vi "SLM_Camera_Rotatory_MAIN_v2.vi"() -> ()   [LabVIEW 2025]
uses:
  LabVIEW_utils_nick/hologram_states.ctl
  LabVIEW_utils_nick/rotatory_motor_states.ctl
  LabVIEW_utils_nick/states_camera.ctl
panel:
  in  "Fine Tune\nPhase (deg)":dbl=-48.0
  in  "Defocus (mm)":dbl step=1.0
  out "Camera State Queue":refnum<queue>
  out "Motor State Queue":refnum<queue>
  out "SLM State Queue":refnum<queue>
  out "Signal Ready":bool=TRUE
  in  "Pupil Diam. (mm)":dbl=5.6
  in  "Linear Period Y":dbl
  in  "Linear Period X":dbl=-16.0
  in  "SLM Correction":string(combo)="Double-Pass Correction"
  in  "Multipurpose\nCoefficient":dbl
  in  "Eff. Pixel Size":dbl=4.0 step=0.01
  in  "Astigmatism (l)":dbl step=0.01
  in  "Degree Sampling":dbl=1.0
  in  "Calibrate QWP":bool
  in  "N Angles":i16=8 min=8 max=200 step=2
  in  "Measure Stokes":bool
  out "Motor Ready":bool
  in  "Disconnect Motor":bool
  in  "Backward":bool
  in  "Forward":bool
  in  "Motor Name":string="0"
  in  "Encoder Steps/º":i32=398
  in  "Jog Angle (º)":dbl=22.5 format="%#_13g"
  in  "VISA Rotatory Motor":refnum<visa-resource-name>="COM4"
  in  "Connect Motor":bool
  out "SLM Ready":bool=TRUE
  in  "Connect Camera":bool
  in  "View Tab":T1(tab)=enum."Camera Live View"
  out "SLM Display":T2(plugin-control)
  in  "ICImagingControl":refnum<k7>(container)
  out "Snapped Image":T2(plugin-control)
  out "LUT Graph":cluster{dbl[], dbl[]}(graph)={[0.0, 1.0, 2.0, 3.0, 4.0, 5.0, 6.0, 7.0, 8.0, 9.0, 10.0, 11.0, 12.0, 13.0, 14.0, 15.0, 16.0, 17.0, 18.0, 19.0, 20.0, 21.0, 22.0, 23.0, 24.0, 25.0, 26.0, 27.0, 28.0, 29.0, 30.0, 31.0, 32.0, 33.0, 34.0, 35.0, 36.0, 37.0, 38.0, 39.0, 40.0, 41.0, 42.0, 43.0, 44.0, 45.0, 46.0, 47.0, 48.0, 49.0, 50.0, 51.0, 52.0, 53.0, 54.0, 55.0, 56.0, 57.0, 58.0, 59.0, 60.0, 61.0, 62.0, 63.0, 64.0, 65.0, 66.0, 67.0, 68.0, 69.0, 70.0, 71.0, 72.0, 73.0, 74.0, 75.0, 76.0, 77.0, 78.0, 79.0, 80.0, 81.0, 82.0, 83.0, 84.0, 85.0, 86.0, 87.0, 88.0, 89.0, 90.0, 91.0, 92.0, 93.0, 94.0, 95.0, 96.0, 97.0, 98.0, 99.0, 100.0, 101.0, 102.0, 103.0, 104.0, 105.0, 106.0, 107.0, 108.0, 109.0, 110.0, 111.0, 112.0, 113.0, 114.0, 115.0, 116.0, 117.0, 118.0, 119.0, 120.0, 121.0, 122.0, 123.0, 124.0, 125.0, 126.0, 127.0, 128.0, 129.0, 130.0, 131.0, 132.0, 133.0, 134.0, 135.0, 136.0, 137.0, 138.0, 139.0, 140.0, 141.0, 142.0, 143.0, 144.0, 145.0, 146.0, 147.0, 148.0, 149.0, 150.0, 151.0, 152.0, 153.0, 154.0, 155.0, 156.0, 157.0, 158.0, 159.0, 160.0, 161.0, 162.0, 163.0, 164.0, 165.0, 166.0, 167.0, 168.0, 169.0, 170.0, 171.0, 172.0, 173.0, 174.0, 175.0, 176.0, 177.0, 178.0, 179.0, 180.0, 181.0, 182.0, 183.0, 184.0, 185.0, 186.0, 187.0, 188.0, 189.0, 190.0, 191.0, 192.0, 193.0, 194.0], [0.0, 0.010256410256410256, 0.020512820512820513, 0.030769230769230767, 0.041025641025641026, 0.05128205128205128, 0.061538461538461535, 0.07179487179487179, 0.08205128205128205, 0.0923076923076923, 0.10256410256410256, 0.11282051282051282, 0.12307692307692307, 0.13333333333333333, 0.14358974358974358, 0.15384615384615383, 0.1641025641025641, 0.17435897435897432, 0.1846153846153846, 0.19487179487179487, 0.20512820512820512, 0.21538461538461537, 0.22564102564102564, 0.2358974358974359, 0.24615384615384614, 0.2564102564102564, 0.26666666666666666, 0.27692307692307694, 0.28717948717948716, 0.2974358974358974, 0.30769230769230765, 0.31794871794871793, 0.3282051282051282, 0.3384615384615384, 0.34871794871794864, 0.358974358974359, 0.3692307692307692, 0.37948717948717947, 0.38974358974358975, 0.4, 0.41025641025641024, 0.42051282051282046, 0.43076923076923074, 0.441025641025641, 0.4512820512820513, 0.4615384615384615, 0.4717948717948718, 0.48205128205128206, 0.4923076923076923, 0.5025641025641026, 0.5128205128205128, 0.5230769230769231, 0.5333333333333333, 0.5435897435897435, 0.5538461538461539, 0.5641025641025641, 0.5743589743589743, 0.5846153846153845, 0.5948717948717948, 0.6051282051282051, 0.6153846153846153, 0.6256410256410256, 0.6358974358974359, 0.6461538461538462, 0.6564102564102564, 0.6666666666666666, 0.6769230769230768, 0.6871794871794871, 0.6974358974358973, 0.7076923076923077, 0.717948717948718, 0.7282051282051282, 0.7384615384615384, 0.7487179487179487, 0.7589743589743589, 0.7692307692307692, 0.7794871794871795, 0.7897435897435897, 0.8, 0.8102564102564103, 0.8205128205128205, 0.8307692307692307, 0.8410256410256409, 0.8512820512820511, 0.8615384615384615, 0.8717948717948718, 0.882051282051282, 0.8923076923076922, 0.9025641025641026, 0.9128205128205128, 0.923076923076923, 0.9333333333333332, 0.9435897435897436, 0.9538461538461539, 0.9641025641025641, 0.9743589743589743, 0.9846153846153846, 0.9948717948717948, 1.005128205128205, 1.0153846153846153, 1.0256410256410255, 1.035897435897436, 1.0461538461538462, 1.0564102564102564, 1.0666666666666667, 1.0769230769230769, 1.087179487179487, 1.0974358974358973, 1.1076923076923078, 1.117948717948718, 1.1282051282051282, 1.1384615384615384, 1.1487179487179486, 1.1589743589743589, 1.169230769230769, 1.1794871794871793, 1.1897435897435895, 1.2, 1.2102564102564102, 1.2205128205128204, 1.2307692307692306, 1.241025641025641, 1.2512820512820513, 1.2615384615384615, 1.2717948717948717, 1.282051282051282, 1.2923076923076924, 1.3025641025641024, 1.3128205128205128, 1.323076923076923, 1.3333333333333333, 1.3435897435897437, 1.3538461538461537, 1.3641025641025641, 1.3743589743589741, 1.3846153846153846, 1.3948717948717946, 1.405128205128205, 1.4153846153846155, 1.4256410256410255, 1.435897435897436, 1.446153846153846, 1.4564102564102563, 1.4666666666666666, 1.4769230769230768, 1.4871794871794872, 1.4974358974358974, 1.5076923076923077, 1.5179487179487179, 1.528205128205128, 1.5384615384615383, 1.5487179487179488, 1.558974358974359, 1.5692307692307692, 1.5794871794871794, 1.5897435897435896, 1.6, 1.61025641025641, 1.6205128205128205, 1.6307692307692305, 1.641025641025641, 1.6512820512820514, 1.6615384615384614, 1.6717948717948719, 1.6820512820512818, 1.6923076923076923, 1.7025641025641023, 1.7128205128205127, 1.723076923076923, 1.7333333333333332, 1.7435897435897436, 1.7538461538461536, 1.764102564102564, 1.7743589743589743, 1.7846153846153845, 1.7948717948717947, 1.8051282051282052, 1.8153846153846154, 1.8256410256410256, 1.8358974358974358, 1.846153846153846, 1.8564102564102565, 1.8666666666666665, 1.876923076923077, 1.8871794871794871, 1.8974358974358974, 1.9076923076923078, 1.9179487179487178, 1.9282051282051282, 1.9384615384615382, 1.9487179487179487, 1.9589743589743587, 1.9692307692307691, 1.9794871794871796, 1.9897435897435896]}
  out "?":cluster{dbl[], dbl[]}(graph)={[0.0, 1.0, 2.0, 3.0, 4.0, 5.0, 6.0, 7.0, 8.0, 9.0, 10.0, 11.0, 12.0, 13.0, 14.0, 15.0, 16.0, 17.0, 18.0, 19.0, 20.0, 21.0, 22.0, 23.0, 24.0, 25.0, 26.0, 27.0, 28.0, 29.0, 30.0, 31.0, 32.0, 33.0, 34.0, 35.0, 36.0, 37.0, 38.0, 39.0, 40.0, 41.0, 42.0, 43.0, 44.0, 45.0, 46.0, 47.0, 48.0, 49.0, 50.0, 51.0, 52.0, 53.0, 54.0, 55.0, 56.0, 57.0, 58.0, 59.0, 60.0, 61.0, 62.0, 63.0, 64.0, 65.0, 66.0, 67.0, 68.0, 69.0, 70.0, 71.0, 72.0, 73.0, 74.0, 75.0, 76.0, 77.0, 78.0, 79.0, 80.0, 81.0, 82.0, 83.0, 84.0, 85.0, 86.0, 87.0, 88.0, 89.0], [4633679.0, 4655841.0, 4685689.0, 4715698.0, 4744099.0, 4772883.0, 4798670.0, 4826914.0, 4870347.0, 4902083.0, 4922698.0, 4948098.0, 4972552.0, 4995565.0, 5012827.0, 5039209.0, 5052894.0, 5073829.0, 5095346.0, 5114978.0, 5130238.0, 5145058.0, 5165064.0, 5171724.0, 5186128.0, 5187223.0, 5193101.0, 5193411.0, 5194593.0, 5192009.0, 5190420.0, 5184407.0, 5176882.0, 5173530.0, 5161350.0, 5144839.0, 5116936.0, 5111336.0, 5101183.0, 5084166.0, 5070283.0, 5047925.0, 5026346.0, 4999847.0, 4976683.0, 4951600.0, 4928131.0, 4900049.0, 4877127.0, 4851185.0, 4827069.0, 4802488.0, 4781082.0, 4752465.0, 4728072.0, 4703937.0, 4678367.0, 4654771.0, 4629539.0, 4610946.0, 4587405.0, 4565992.0, 4549223.0, 4538346.0, 4521123.0, 4508564.0, 4497075.0, 4492614.0, 4476652.0, 4467015.0, 4463359.0, 4461451.0, 4458074.0, 4459501.0, 4457195.0, 4462532.0, 4470243.0, 4474909.0, 4478224.0, 4493369.0, 4502945.0, 4519712.0, 4534878.0, 4551381.0, 4567135.0, 4590315.0, 4609051.0, 4633947.0, 4651470.0, 4667315.0]}
  in  "Live":bool
  in  "Disconnect Camera":bool
  in  "Camera Properties":bool
  out "Camera Ready":bool
  in  "Grab Image":bool
  in  "Send to SLM":bool=TRUE
  in  "Stop All":bool
  in  "Laser Line (nm)":i32=488
  in  "SLM Cols":i32=1280
  in  "SLM Rows":i32=1024
  in  "Modulation Tab":enum32{"Double Pass", "Single Pass"}(tab)
  in  "Y Offset B":i32 step=1
  in  "Y Offset A":i32 step=1
  in  "X Offset A":i32 step=1
  in  "B Display (Ex)":bool=TRUE
  in  "A Display (Ey)":bool=TRUE
  in  "X Offset B":i32 step=1
  in  "Modulation Mode Double Pass":string(combo)="Laguerre-Gaussian Left"
  in  "Y Offset":i32
  in  "X Offset":i32
  in  "Modulation Type Single Pass":string(combo)="Arrizon Test"
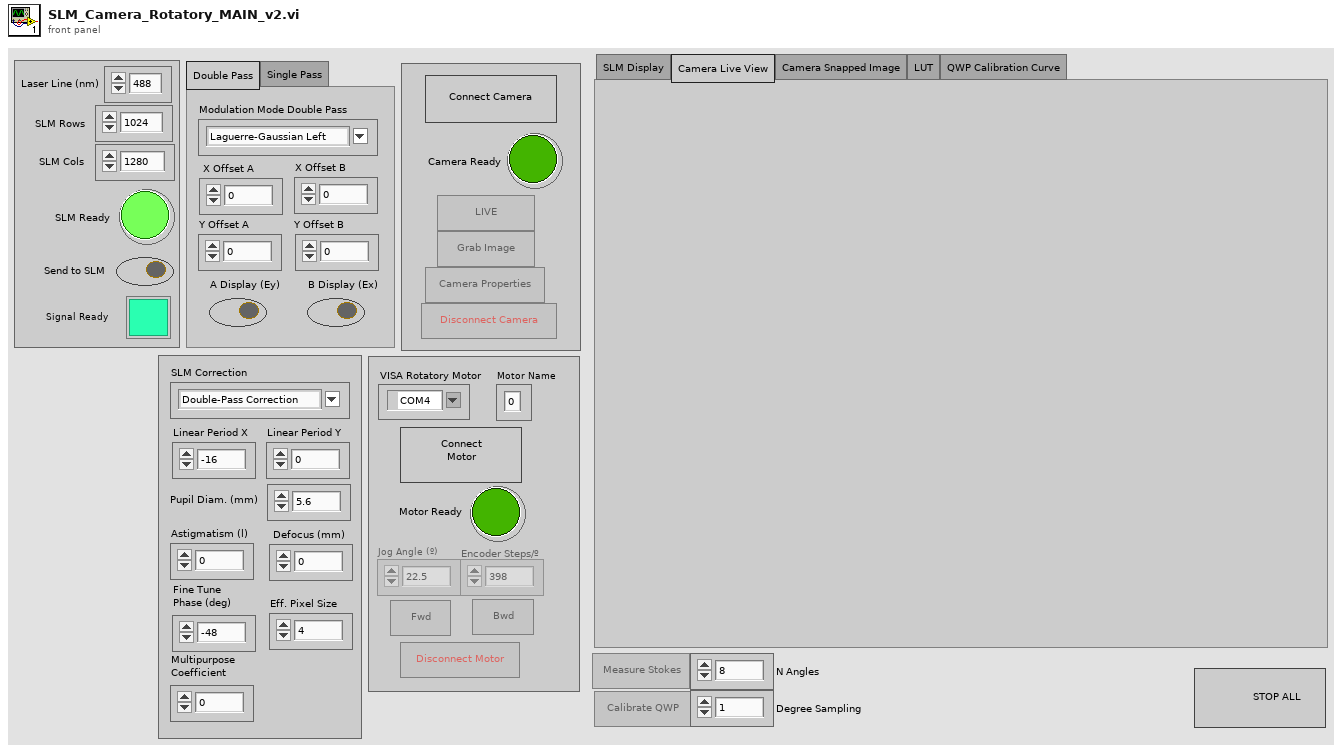
[diagram p1: front panel]
types:
  T1 = enum32{"SLM Display", "Camera Live View", "Camera Snapped Image", "LUT", "QWP Calibration Curve"}
  T2 = typedef "IMAQ Image.ctl" = refnum<image>
  T3 = typedef "rotatory_motor_states.ctl" = enum16{"Set Jog Step", "Move Forward", "Disconnect Motor", "Connect Motor", "Stop All", "Move Backward", "Idle"}
  T4 = typedef "states_camera.ctl" = enum16{"Calibrate QWP Position", "Measure Stokes", "Init Camera", "Idle", "Open Properties", "Grab Image", "Disconnect Camera", "Set Live", "Stop Program", "Calibrate SLM Phase Modulation"}
  T5 = typedef "hologram_states.ctl" = enum16{"Init", "Idle", "Compute Modulation", "Stop All", "Send to SLM"}
  T6 = enum16{"Init", "Idle", "Compute Modulation", "Stop All"}
  T7 = cluster{"status":bool, "code":bool, "source":bool}
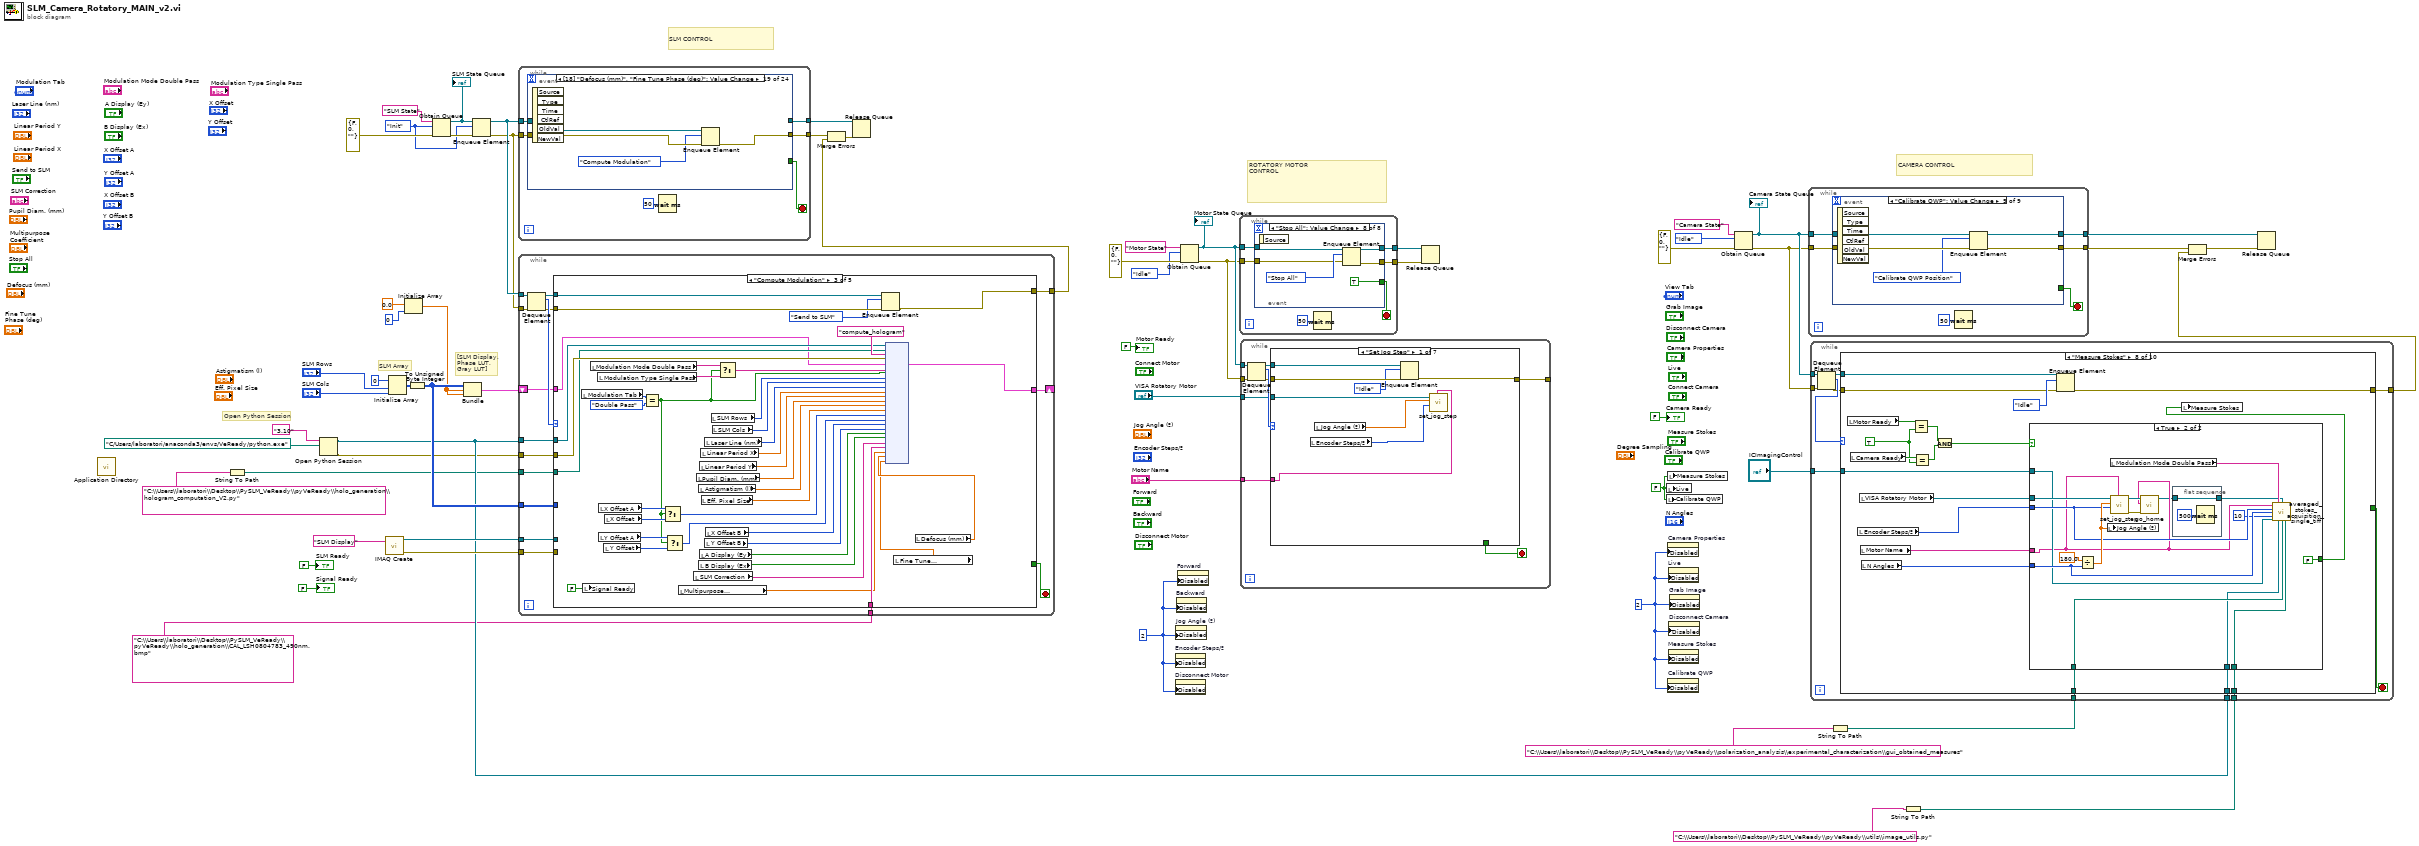
[diagram p0: block diagram]
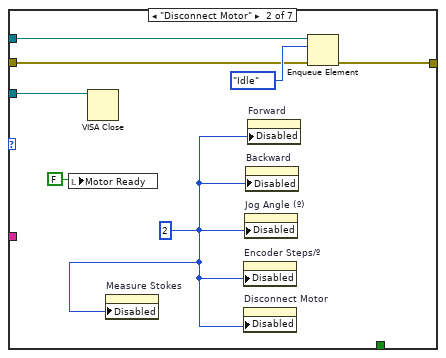
[diagram p2: hidden frame]
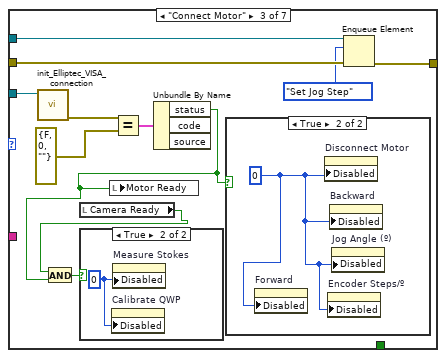
[diagram p3: hidden frame]
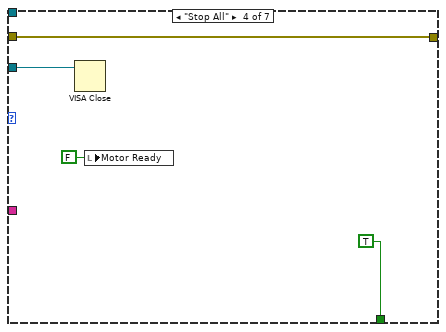
[diagram p6: hidden frame]
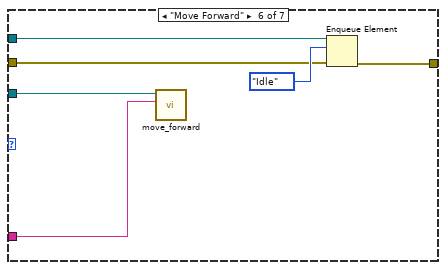
[diagram p8: hidden frame]
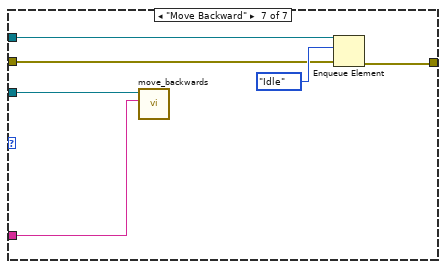
[diagram p9: hidden frame]
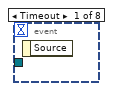
[diagram p10: hidden frame]
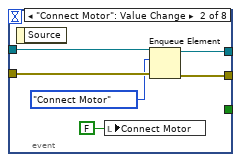
[diagram p11: hidden frame]
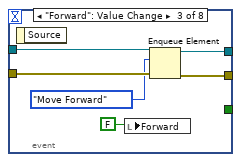
[diagram p12: hidden frame]
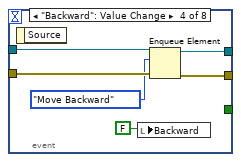
[diagram p13: hidden frame]
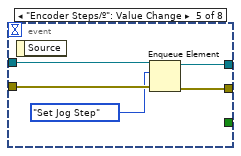
[diagram p14: hidden frame]
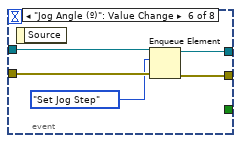
[diagram p15: hidden frame]
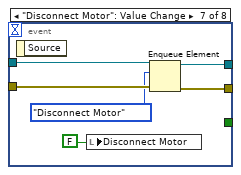
[diagram p16: hidden frame]
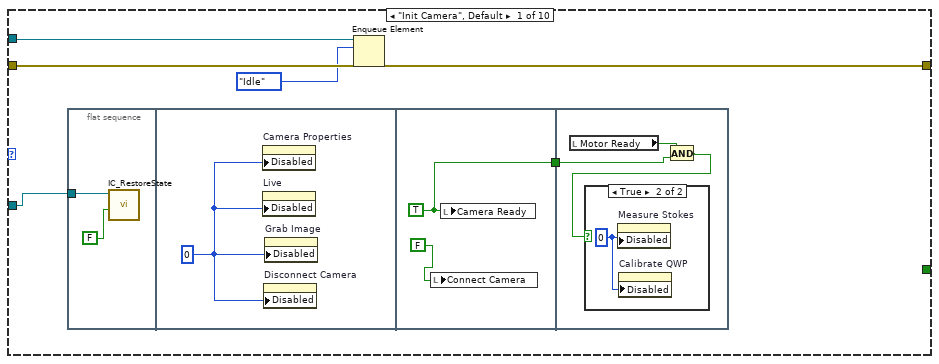
[diagram p17: hidden frame]
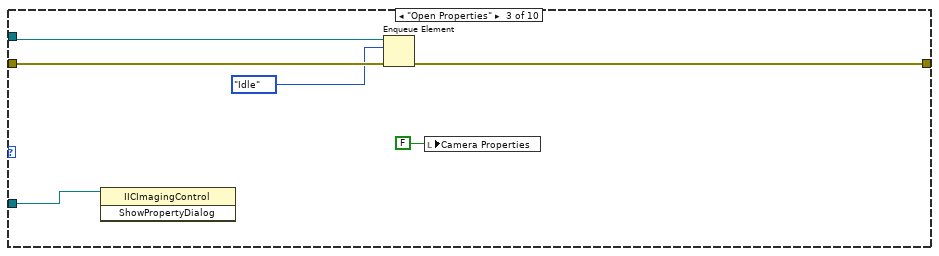
[diagram p20: hidden frame]
diagram:
  w26 = u8 2 ("Disabled")
  w18 = FALSE
  w19 = u8 2 ("Disabled")
  w47 = hologram_states."Init"
  # "Open Python Session"
  # "[SLM Display,\nPhase LUT,\nGray LUT]"
  # "SLM Array"
  # "ROTATORY MOTOR\nCONTROL"
  # "CAMERA CONTROL"
  # "SLM CONTROL"
  n1 = call <vilib>:"Application Directory.vi"() -> ()  [unwired: 1 out]
  n2 = String To Path(string="C:\\Users\\laboratori\\Desktop\\PySLM_VeReady\\pyVeReady\\holo_generation\\hologram_computation_V2.py") -> (path=w7:path)
  n3 = Open Python Session(python version="3.10" ("Python version"), python path=path "C:/Users/laboratori/anaconda3/envs/VeReady/python.exe" ("Python path")) -> (session out=w9:refnum<k35>, error out=w8:errorcluster)  [unwired: 1 in]
  n4 = call "IMAQ Create"("Image Name"="SLM Display") -> ("New Image"=w53:T2, "error out"=w52:errorcluster)  [unwired: 4 in]
  n5 = Initialize Array(0, "SLM Rows", "SLM Cols") -> (w24:i32[][])
  n6 = Initialize Array(0.0, 0 ("dimension size")) -> (w13:dbl[])
  n7 = To Unsigned Byte Integer(number=w24) -> (unsigned 8bit integer=w16:u8[][])
  n8 = Obtain Queue(name (unnamed)="SLM State", element data type=w47, error in (no error)=errorcluster {"status"=FALSE, "code"=0, "source"=""}) -> (queue out=w51:refnum<queue>, error out=w49:errorcluster)  [unwired: 2 in, 1 out]
  "SLM State Queue" <- w51
  n9 = Bundle(w16, w13, w13) -> (w12:cluster{u8[][], dbl[], dbl[]})  [unwired: 1 in]
  n10 = Enqueue Element(queue=w51, element=w47, error in (no error)=w49) -> (queue out=w50:refnum<queue>, error out=w48:errorcluster)  [unwired: 1 in, 1 out]
  n11 = while {
    tunnel: w50 -> [w64]
    tunnel: [w63] -> w59
    tunnel: [w62] -> w57
    tunnel: w48 -> [w61]
    stop <- w65 stop-if-true
    n12 = event shown="[18] \"Defocus (mm)\", \"Fine Tune Phase (deg)\": Value Change" {
      selector: _ -> [_ _ _ _ _ _ _ _ _ _ _ _ _ _ _ _ _ _ _ _ _ _ _ _]
      dyn-events: _ -> [_ _ _ _ _ _ _ _ _ _ _ _ _ _ _ _ _ _ _ _ _ _ _ _]
      timeout: _ -> [_ _ _ _ _ _ _ _ _ _ _ _ _ _ _ _ _ _ _ _ _ _ _ _]
      tunnel: [_ _ _ _ _ _ _ _ _ _ _ _ _ _ _ _ _ _ _ _ _ TRUE _ _] -> w65
      tunnel: w64 -> [_ w71 w76 w81 w86 w91 w96 w101 w106 w111 w116 w121 w126 w131 w136 w140 w144 w148 w152 w156 w160 w166 w172 w177]
      tunnel: [_ w70 w75 w80 w85 w90 w95 w100 w105 w110 w115 w120 w125 w130 w135 _ _ _ _ _ _ w163 w171 w176] -> w63
      tunnel: [_ w69 w74 w79 w84 w89 w94 w99 w104 w109 w114 w119 w124 w129 w134 w138 w142 w146 w150 w154 w158 w164 w169 w174] -> w62
      tunnel: w61 -> [_ w67 w72 w77 w82 w87 w92 w97 w102 w107 w112 w117 w122 w127 w132 w139 w143 w147 w151 w155 w159 w165 w170 w175]
      event Timeout {
        n13 = event-data() -> ()  [unwired: 1 in, 3 out]
      }
      event "Modulation Mode Double Pass": Value Change {
        n14 = event-data() -> ()  [unwired: 1 in, 1 out]
        n15 = Enqueue Element(queue=w71, element=enum16{"Init", "Idle", "Compute Modulation"}."Compute Modulation", error in (no error)=w67) -> (queue out=w70:refnum<queue>, error out=w69:errorcluster)  [unwired: 1 in, 1 out]
      }
      event "Laser Line (nm)": Value Change {
        n16 = event-data() -> ()  [unwired: 1 in, 1 out]
        n17 = Enqueue Element(queue=w76, element=enum16{"Init", "Idle", "Compute Modulation"}."Compute Modulation", error in (no error)=w72) -> (queue out=w75:refnum<queue>, error out=w74:errorcluster)  [unwired: 1 in, 1 out]
      }
      event "Astigmatism (l)": Value Change {
        n18 = event-data() -> ()  [unwired: 1 in, 6 out]
        n19 = Enqueue Element(queue=w81, element=enum16{"Init", "Idle", "Compute Modulation"}."Compute Modulation", error in (no error)=w77) -> (queue out=w80:refnum<queue>, error out=w79:errorcluster)  [unwired: 1 in, 1 out]
      }
      event "Eff. Pixel Size": Value Change {
        n20 = event-data() -> ()  [unwired: 1 in, 6 out]
        n21 = Enqueue Element(queue=w86, element=enum16{"Init", "Idle", "Compute Modulation"}."Compute Modulation", error in (no error)=w82) -> (queue out=w85:refnum<queue>, error out=w84:errorcluster)  [unwired: 1 in, 1 out]
      }
      event "Linear Period X": Value Change {
        n22 = event-data() -> ()  [unwired: 1 in, 1 out]
        n23 = Enqueue Element(queue=w91, element=enum16{"Init", "Idle", "Compute Modulation"}."Compute Modulation", error in (no error)=w87) -> (queue out=w90:refnum<queue>, error out=w89:errorcluster)  [unwired: 1 in, 1 out]
      }
      event "Pupil Diam. (mm)": Value Change {
        n24 = event-data() -> ()  [unwired: 1 in, 6 out]
        n25 = Enqueue Element(queue=w96, element=enum16{"Init", "Idle", "Compute Modulation"}."Compute Modulation", error in (no error)=w92) -> (queue out=w95:refnum<queue>, error out=w94:errorcluster)  [unwired: 1 in, 1 out]
      }
      event "SLM Correction": Value Change {
        n26 = event-data() -> ()  [unwired: 1 in, 6 out]
        n27 = Enqueue Element(queue=w101, element=enum16{"Init", "Idle", "Compute Modulation"}."Compute Modulation", error in (no error)=w97) -> (queue out=w100:refnum<queue>, error out=w99:errorcluster)  [unwired: 1 in, 1 out]
      }
      event "Linear Period Y": Value Change {
        n28 = event-data() -> ()  [unwired: 1 in, 1 out]
        n29 = Enqueue Element(queue=w106, element=enum16{"Init", "Idle", "Compute Modulation"}."Compute Modulation", error in (no error)=w102) -> (queue out=w105:refnum<queue>, error out=w104:errorcluster)  [unwired: 1 in, 1 out]
      }
      event "SLM Rows": Value Change {
        n30 = event-data() -> ()  [unwired: 1 in, 1 out]
        n31 = Enqueue Element(queue=w111, element=enum16{"Init", "Idle", "Compute Modulation"}."Compute Modulation", error in (no error)=w107) -> (queue out=w110:refnum<queue>, error out=w109:errorcluster)  [unwired: 1 in, 1 out]
      }
      event "Multipurpose\nCoefficient": Value Change {
        n32 = event-data() -> ()  [unwired: 1 in, 6 out]
        n33 = Enqueue Element(queue=w116, element=enum16{"Init", "Idle", "Compute Modulation"}."Compute Modulation", error in (no error)=w112) -> (queue out=w115:refnum<queue>, error out=w114:errorcluster)  [unwired: 1 in, 1 out]
      }
      event "Modulation Type Single Pass": Value Change {
        n34 = event-data() -> ()  [unwired: 1 in, 6 out]
        n35 = Enqueue Element(queue=w121, element=enum16{"Init", "Idle", "Compute Modulation"}."Compute Modulation", error in (no error)=w117) -> (queue out=w120:refnum<queue>, error out=w119:errorcluster)  [unwired: 1 in, 1 out]
      }
      event "X Offset": Value Change {
        n36 = event-data() -> ()  [unwired: 1 in, 6 out]
        n37 = Enqueue Element(queue=w126, element=enum16{"Init", "Idle", "Compute Modulation"}."Compute Modulation", error in (no error)=w122) -> (queue out=w125:refnum<queue>, error out=w124:errorcluster)  [unwired: 1 in, 1 out]
      }
      event "Y Offset": Value Change {
        n38 = event-data() -> ()  [unwired: 1 in, 6 out]
        n39 = Enqueue Element(queue=w131, element=enum16{"Init", "Idle", "Compute Modulation"}."Compute Modulation", error in (no error)=w127) -> (queue out=w130:refnum<queue>, error out=w129:errorcluster)  [unwired: 1 in, 1 out]
      }
      event "SLM Cols": Value Change {
        n40 = event-data() -> ()  [unwired: 1 in, 1 out]
        n41 = Enqueue Element(queue=w136, element=enum16{"Init", "Idle", "Compute Modulation"}."Compute Modulation", error in (no error)=w132) -> (queue out=w135:refnum<queue>, error out=w134:errorcluster)  [unwired: 1 in, 1 out]
      }
      event "X Offset A": Value Change {
        n42 = event-data() -> ()  [unwired: 1 in, 1 out]
        n43 = Enqueue Element(queue=w140, element=hologram_states."Compute Modulation", error in (no error)=w139) -> (error out=w138:errorcluster)  [unwired: 1 in, 2 out]
      }
      event "Send to SLM": Value Change {
        n44 = event-data() -> ()  [unwired: 1 in, 1 out]
        n45 = Enqueue Element(queue=w144, element=hologram_states."Send to SLM", error in (no error)=w143) -> (error out=w142:errorcluster)  [unwired: 1 in, 2 out]
      }
      event "Y Offset A": Value Change {
        n46 = event-data() -> ()  [unwired: 1 in, 1 out]
        n47 = Enqueue Element(queue=w148, element=hologram_states."Compute Modulation", error in (no error)=w147) -> (error out=w146:errorcluster)  [unwired: 1 in, 2 out]
      }
      event "Defocus (mm)", "Fine Tune\nPhase (deg)": Value Change {
        n48 = event-data() -> ()  [unwired: 1 in, 6 out]
        n49 = Enqueue Element(queue=w152, element=hologram_states."Compute Modulation", error in (no error)=w151) -> (error out=w150:errorcluster)  [unwired: 1 in, 2 out]
      }
      event "X Offset B": Value Change {
        n50 = event-data() -> ()  [unwired: 1 in, 1 out]
        n51 = Enqueue Element(queue=w156, element=hologram_states."Compute Modulation", error in (no error)=w155) -> (error out=w154:errorcluster)  [unwired: 1 in, 2 out]
      }
      event "Y Offset B": Value Change {
        n52 = event-data() -> ()  [unwired: 1 in, 1 out]
        n53 = Enqueue Element(queue=w160, element=hologram_states."Compute Modulation", error in (no error)=w159) -> (error out=w158:errorcluster)  [unwired: 1 in, 2 out]
      }
      event "Stop All": Value Change {
        n54 = event-data() -> ()  [unwired: 1 in, 1 out]
        n55 = local write "Stop All"(FALSE) -> ()
        n56 = Enqueue Element(queue=w166, element=T6."Stop All", error in (no error)=w165) -> (queue out=w163:refnum<queue>, error out=w164:errorcluster)  [unwired: 1 in, 1 out]
      }
      event "A Display (Ey)": Value Change {
        n57 = event-data() -> ()  [unwired: 1 in, 1 out]
        n58 = Enqueue Element(queue=w172, element=hologram_states."Compute Modulation", error in (no error)=w170) -> (queue out=w171:refnum<queue>, error out=w169:errorcluster)  [unwired: 1 in, 1 out]
      }
      event "B Display (Ex)": Value Change {
        n59 = event-data() -> ()  [unwired: 1 in, 1 out]
        n60 = Enqueue Element(queue=w177, element=hologram_states."Compute Modulation", error in (no error)=w175) -> (queue out=w176:refnum<queue>, error out=w174:errorcluster)  [unwired: 1 in, 1 out]
      }
    }
    n61 = Wait (ms)(milliseconds to wait=u32 50) -> ()  [unwired: 1 out]
  }
  n62 = while {
    tunnel: w50 -> [w193]
    tunnel: w48 -> [w192]
    tunnel: [w190] -> w58
    tunnel: w9 -> [w187]
    tunnel: w8 -> [w186]
    tunnel: w7 -> [w185]
    tunnel: w53 -> [w183]
    tunnel: w52 -> [w182]
    shift-right: [w180] -> _
    shift-left: w12 -> [w179]
    tunnel: w16 -> [w181]
    tunnel: "C:\\Users\\laboratori\\Desktop\\PySLM_VeReady\\pyVeReady\\holo_generation\\CAL_LSH0804783_490nm.bmp" -> [w178]
    stop <- w188 stop-if-true
    n63 = Dequeue Element(queue=w193, error in (no error)=w192) -> (queue out=w184:refnum<queue>, element=w191:T5, error out=w189:errorcluster)  [unwired: 1 in, 1 out]
    n64 = case shown="\"Compute Modulation\"" w191 {
      tunnel: [w218 _ w259 _ w277] -> w190
      tunnel: w189 -> [w220 _ w261 _ w278]
      tunnel: [_ _ _ TRUE _] -> w188
      tunnel: w187 -> [w217 _ w249 w269 _]
      tunnel: w186 -> [w216 _ w248 w268 _]
      tunnel: w185 -> [w215 _ w247 _ _]
      tunnel: w184 -> [w219 _ w260 _ w279]
      tunnel: w183 -> [w213 _ _ w267 w285]
      tunnel: w182 -> [w212 _ _ w266 w284]
      tunnel: w181 -> [_ _ _ _ w281]
      tunnel: [w194 w222 w237 w263 w275] -> w180
      tunnel: w179 -> [w194 w222 w238 w263 w275]
      tunnel: w178 -> [_ _ w239 _ _]
      frame "Init" {
        w199 = errorcluster {"status"=FALSE, "code"=0, "source"=""} ("y")
        w210 = TRUE ("Window has title bar? (Yes)")
        w209 = FALSE ("Window has title bar? (Yes)")
        w208 = 0 ("Window Number (0...15)")
        # "Send Zeros to Display"
        n65 = local write "Modulation Mode Double Pass"("") -> ()
        n66 = node(w217, w215, "dummy_function" ("function name"), w216) -> (w201:errorcluster)  [unwired: 2 in, 3 out]
        n67 = call "IMAQ ArrayToImage"("error in (no error)"=w212, "Image"=w213) -> ("error out"=w204:errorcluster, "Image Out"=w203:T2)  [unwired: 8 in]
        "SLM Display" <- w203
        n68 = Equal?(x=w201, y=w199) -> (x = y?=w198:T7)
        n69 = call "IMAQ WindSetup"("Window is floating? (No)"=w210, "Window Number (0...15)"=w208, "error in (no error)"=w204, "Window has title bar? (Yes)"=w209, "Window can grow? (Yes)"=w209) -> ("error out"=w211:errorcluster)  [unwired: 6 in]
        n70 = call "IMAQ WindShow"("error in (no error)"=w211, "Bring To Front? (N)"=w210, "Hide/Show (Show)"=w210, "Window Number (0...15)"=w208) -> ("error out"=w205:errorcluster)  [unwired: 2 in, 2 out]
        n71 = call "IMAQ WindDraw"("Window Number (0...15)"=w208, "error in (no error)"=w205, "Image"=w203) -> ("error out"=w206:errorcluster)  [unwired: 7 in, 1 out]
        n72 = call "IMAQ WindMove"("Window Number (0...15)"=w208, "Coordinates (screen)"=cluster{"X Position":i32, "Y Position":i32} {"X Position"=2560, "Y Position"=0}, "error in (no error)"=w206) -> ("error out"=w200:errorcluster)  [unwired: 2 in, 1 out]
        n73 = Enqueue Element(queue=w219, element=T6."Idle", error in (no error)=w220) -> (error out=w218:errorcluster)  [unwired: 1 in, 2 out]
        n74 = Equal?(x=w199, y=w200) -> (x = y?=w197:T7)
        n75 = And(x=w198, y=w197) -> (x .and. y?=w196:T7)
        n76 = Unbundle(w196) -> ("status"=w195:bool)  [unwired: 2 out]
        n77 = local write "SLM Ready"(w195) -> ()
      }
      frame "Idle", Default {
      }
      frame "Compute Modulation" {
        n78 = local read "Modulation Tab"() -> (w258:enum32{"Double Pass", "Single Pass"})
        n79 = local write "Signal Ready"(FALSE) -> ()
        n80 = local read "Modulation Mode Double Pass"() -> (w235:string)
        n81 = local read "Modulation Type Single Pass"() -> (w234:string)
        n82 = local read "X Offset A"() -> (w232:i32)
        n83 = local read "Y Offset A"() -> (w229:i32)
        n84 = local read "Y Offset"() -> (w228:i32)
        n85 = local read "X Offset"() -> (w231:i32)
        n86 = Equal?(x=w258, y=enum32{"Double Pass", "Single Pass"}."Double Pass") -> (x = y?=w227:bool)
        n87 = Select(t=w232, s=w227, f=w231) -> (s? t:f=w230:i32)
        n88 = Select(t=w229, s=w227, f=w228) -> (s? t:f=w226:i32)
        n89 = local read "Multipurpose\nCoefficient"() -> (w236:dbl)
        n90 = local read "SLM Correction"() -> (w240:string)
        n91 = local read "Pupil Diam. (mm)"() -> (w251:dbl)
        n92 = local read "Astigmatism (l)"() -> (w246:dbl)
        n93 = local read "B Display (Ex)"() -> (w241:bool)
        n94 = local read "Linear Period Y"() -> (w252:dbl)
        n95 = local read "A Display (Ey)"() -> (w242:bool)
        n96 = local read "Linear Period X"() -> (w253:dbl)
        n97 = local read "Eff. Pixel Size"() -> (w245:dbl)
        n98 = local read "Laser Line (nm)"() -> (w254:i32)
        n99 = local read "Y Offset B"() -> (w243:i32)
        n100 = local read "X Offset B"() -> (w244:i32)
        n101 = local read "SLM Rows"() -> (w256:i32)
        n102 = local read "SLM Cols"() -> (w255:i32)
        n103 = Select(t=w235, s=w227, f=w234) -> (s? t:f=w233:string)
        n104 = Enqueue Element(queue=w260, element=hologram_states."Send to SLM", error in (no error)=w261) -> (error out=w259:errorcluster)  [unwired: 1 in, 2 out]
        n105 = local read "Fine Tune\nPhase (deg)"() -> (w223:dbl)
        n106 = local read "Defocus (mm)"() -> (w224:dbl)
        n107 = node(w249, w247, "compute_hologram" ("function name"), w248, w238, w233, w227, w256, w255, w254, w253, w252, w251, w246, w245, w230, w226, w244, w243, w242, w241, w240, w239, w236, w224, w223) -> (w237:cluster{u8[][], dbl[], dbl[]})  [unwired: 21 in, 4 out]
      }
      frame "Stop All" {
        n108 = local write "SLM Ready"(FALSE) -> ()
        n109 = call "IMAQ Dispose"("Image"=w267, "error in (no error)"=w266) -> ()  [unwired: 1 in, 4 out]
        n110 = call "IMAQ WindClose"("Window Number (0...15)"=0) -> ()  [unwired: 5 in, 1 out]
        n111 = Close Python Session(session in=w269, error in=w268) -> ()  [unwired: 1 out]
      }
      frame "Send to SLM" {
        n112 = Unbundle(w275) -> (w274:u8[][], w273:dbl[], w272:dbl[])
        n113 = call "IMAQ ArrayToImage"("error in (no error)"=w284, "Image Pixels (U8)"=w274, "Image"=w285) -> ("error out"=w282:errorcluster, "Image Out"=w283:T2)  [unwired: 7 in]
        n114 = Bundle(w272, w273) -> (→"LUT Graph":cluster{dbl[], dbl[]})  [unwired: 1 in]
        n115 = local read "Send to SLM"() -> (w286:bool)
        n116 = local write "SLM Display"(w283) -> ()
        n117 = case shown="False" w286 {
          tunnel: w283 -> [w290 w301]
          tunnel: w282 -> [w289 w300]
          tunnel: w281 -> [w288 _]
          tunnel: [TRUE TRUE] -> w276
          frame False {
            w297 = TRUE ("Window has title bar? (Yes)")
            w296 = FALSE ("Window has title bar? (Yes)")
            w295 = 0 ("Window Number (0...15)")
            n118 = call "IMAQ WindSetup"("Window is floating? (No)"=w297, "Window Number (0...15)"=w295, "error in (no error)"=w289, "Window has title bar? (Yes)"=w296, "Window can grow? (Yes)"=w296) -> ("error out"=w298:errorcluster)  [unwired: 6 in]
            n119 = call "IMAQ ArrayToImage"("Image Pixels (U8)"=w288, "Image"=w290) -> ("Image Out"=w291:T2)  [unwired: 8 in, 1 out]
            n120 = call "IMAQ WindShow"("error in (no error)"=w298, "Bring To Front? (N)"=w297, "Hide/Show (Show)"=w297, "Window Number (0...15)"=w295) -> ("error out"=w292:errorcluster)  [unwired: 2 in, 2 out]
            n121 = call "IMAQ WindDraw"("Window Number (0...15)"=w295, "error in (no error)"=w292, "Image"=w291) -> ("error out"=w293:errorcluster)  [unwired: 7 in, 1 out]
            n122 = call "IMAQ WindMove"("Window Number (0...15)"=w295, "Coordinates (screen)"=cluster{"X Position":i32, "Y Position":i32} {"X Position"=2560, "Y Position"=0}, "error in (no error)"=w293) -> ()  [unwired: 2 in, 2 out]
          }
          frame True {
            w307 = TRUE ("Window has title bar? (Yes)")
            w306 = FALSE ("Window has title bar? (Yes)")
            w305 = 0 ("Window Number (0...15)")
            n123 = call "IMAQ WindSetup"("Window is floating? (No)"=w307, "Window Number (0...15)"=w305, "error in (no error)"=w300, "Window has title bar? (Yes)"=w306, "Window can grow? (Yes)"=w306) -> ("error out"=w308:errorcluster)  [unwired: 6 in]
            n124 = call "IMAQ WindShow"("error in (no error)"=w308, "Bring To Front? (N)"=w307, "Hide/Show (Show)"=w307, "Window Number (0...15)"=w305) -> ("error out"=w302:errorcluster)  [unwired: 2 in, 2 out]
            n125 = call "IMAQ WindDraw"("Window Number (0...15)"=w305, "error in (no error)"=w302, "Image"=w301) -> ("error out"=w303:errorcluster)  [unwired: 7 in, 1 out]
            n126 = call "IMAQ WindMove"("Window Number (0...15)"=w305, "Coordinates (screen)"=cluster{"X Position":i32, "Y Position":i32} {"X Position"=2560, "Y Position"=0}, "error in (no error)"=w303) -> ()  [unwired: 2 in, 2 out]
          }
        }
        n127 = Enqueue Element(queue=w279, element=hologram_states."Idle", error in (no error)=w278) -> (error out=w277:errorcluster)  [unwired: 1 in, 2 out]
        n128 = local write "Signal Ready"(w276) -> ()
      }
    }
  }
  n129 = Merge Errors(w57, w58) -> (w56:errorcluster)
  n130 = Release Queue(queue=w59, error in (no error)=w56) -> ()  [unwired: 1 in, 3 out]
  n131 = property on="Encoder Steps/º" class="DigNum (strict)"("Disabled"=w26) -> ()  [unwired: 2 in, 2 out]
  n132 = property on="Disconnect Motor" class="Bool (strict)"("Disabled"=w26) -> ()  [unwired: 2 in, 2 out]
  n133 = property on="Jog Angle (º)" class="DigNum (strict)"("Disabled"=w26) -> ()  [unwired: 2 in, 2 out]
  n134 = property on="Backward" class="Bool (strict)"("Disabled"=w26) -> ()  [unwired: 2 in, 2 out]
  n135 = property on="Forward" class="Bool (strict)"("Disabled"=w26) -> ()  [unwired: 2 in, 2 out]
  n136 = Obtain Queue(name (unnamed)="Motor State", element data type=rotatory_motor_states."Idle", error in (no error)=errorcluster {"status"=FALSE, "code"=0, "source"=""}) -> (queue out=w30:refnum<queue>, error out=w29:errorcluster)  [unwired: 2 in, 1 out]
  "Motor State Queue" <- w30
  n137 = while {
    tunnel: w30 -> [w314]
    tunnel: w29 -> [w313]
    tunnel: [w312] -> w32
    tunnel: [w311] -> w31
    stop <- w309 stop-if-true
    n138 = event shown="[7] \"Stop All\": Value Change" {
      selector: _ -> [_ _ _ _ _ _ _ _]
      dyn-events: _ -> [_ _ _ _ _ _ _ _]
      timeout: _ -> [_ _ _ _ _ _ _ _]
      tunnel: w314 -> [_ w320 w326 w332 w337 w342 w348 w352]
      tunnel: w313 -> [_ w319 w325 w331 w336 w341 w347 w351]
      tunnel: [_ w317 w323 w329 w334 w339 w345 w350] -> w312
      tunnel: [_ w316 w322 w328 w333 w338 w344 w349] -> w311
      tunnel: [_ _ _ _ _ _ _ TRUE] -> w309
      event Timeout {
        n139 = event-data() -> ()  [unwired: 1 in, 1 out]
      }
      event "Connect Motor": Value Change {
        n140 = event-data() -> ()  [unwired: 1 in, 1 out]
        n141 = local write "Connect Motor"(FALSE) -> ()
        n142 = Enqueue Element(queue=w320, element=rotatory_motor_states."Connect Motor", error in (no error)=w319) -> (queue out=w317:refnum<queue>, error out=w316:errorcluster)  [unwired: 1 in, 1 out]
      }
      event "Forward": Value Change {
        n143 = event-data() -> ()  [unwired: 1 in, 1 out]
        n144 = local write "Forward"(FALSE) -> ()
        n145 = Enqueue Element(queue=w326, element=rotatory_motor_states."Move Forward", error in (no error)=w325) -> (queue out=w323:refnum<queue>, error out=w322:errorcluster)  [unwired: 1 in, 1 out]
      }
      event "Backward": Value Change {
        n146 = event-data() -> ()  [unwired: 1 in, 1 out]
        n147 = local write "Backward"(FALSE) -> ()
        n148 = Enqueue Element(queue=w332, element=rotatory_motor_states."Move Backward", error in (no error)=w331) -> (queue out=w329:refnum<queue>, error out=w328:errorcluster)  [unwired: 1 in, 1 out]
      }
      event "Encoder Steps/º": Value Change {
        n149 = event-data() -> ()  [unwired: 1 in, 1 out]
        n150 = Enqueue Element(queue=w337, element=rotatory_motor_states."Set Jog Step", error in (no error)=w336) -> (queue out=w334:refnum<queue>, error out=w333:errorcluster)  [unwired: 1 in, 1 out]
      }
      event "Jog Angle (º)": Value Change {
        n151 = event-data() -> ()  [unwired: 1 in, 1 out]
        n152 = Enqueue Element(queue=w342, element=rotatory_motor_states."Set Jog Step", error in (no error)=w341) -> (queue out=w339:refnum<queue>, error out=w338:errorcluster)  [unwired: 1 in, 1 out]
      }
      event "Disconnect Motor": Value Change {
        n153 = event-data() -> ()  [unwired: 1 in, 1 out]
        n154 = local write "Disconnect Motor"(FALSE) -> ()
        n155 = Enqueue Element(queue=w348, element=rotatory_motor_states."Disconnect Motor", error in (no error)=w347) -> (queue out=w345:refnum<queue>, error out=w344:errorcluster)  [unwired: 1 in, 1 out]
      }
      event "Stop All": Value Change {
        n156 = event-data() -> ()  [unwired: 1 in, 1 out]
        n157 = Enqueue Element(queue=w352, element=rotatory_motor_states."Stop All", error in (no error)=w351) -> (queue out=w350:refnum<queue>, error out=w349:errorcluster)  [unwired: 1 in, 1 out]
      }
    }
    n158 = Wait (ms)(milliseconds to wait=u32 50) -> ()  [unwired: 1 out]
  }
  n159 = while {
    tunnel: w30 -> [w363]
    tunnel: w29 -> [w362]
    tunnel: "VISA Rotatory Motor" -> [w360]
    tunnel: "Motor Name" -> [w358]
    tunnel: [w355] -> _
    stop <- w359 stop-if-true
    n160 = Dequeue Element(queue=w363, error in (no error)=w362) -> (queue out=w357:refnum<queue>, element=w361:T3, error out=w356:errorcluster)  [unwired: 1 in, 1 out]
    n161 = case shown="\"Set Jog Step\"" w361 {
      tunnel: w360 -> [w371 w378 w389 w394 _ w402 w408]
      tunnel: [_ _ _ TRUE _ _ _] -> w359
      tunnel: w358 -> [w364 _ _ _ _ w401 w407]
      tunnel: w357 -> [w370 w376 w388 _ _ w399 w403]
      tunnel: w356 -> [w369 w375 w387 w393 w396 w398 w405]
      tunnel: [w367 w374 w385 w393 w396 w397 w404] -> w355
      frame "Set Jog Step" {
        n162 = local read "Encoder Steps/º"() -> (w365:i32)
        n163 = local read "Jog Angle (º)"() -> (w366:dbl)
        n164 = Enqueue Element(queue=w370, element=rotatory_motor_states."Idle", error in (no error)=w369) -> (error out=w367:errorcluster)  [unwired: 1 in, 2 out]
        n165 = call "set_jog_step.vi"("Motor \"Name\""=w364, "Encoder Pulses per Degree"=w365, "Degrees"=w366, "VISA resource name"=w371) -> ()  [unwired: 5 in, 2 out]
      }
      frame "Disconnect Motor" {
        w372 = u8 2 ("Disabled")
        n166 = local write "Motor Ready"(FALSE) -> ()
        n167 = VISA Close(VISA resource name=w378) -> ()  [unwired: 1 in, 1 out]
        n168 = property on="Measure Stokes" class="Bool (strict)"("Disabled"=w372) -> ()  [unwired: 2 in, 2 out]
        n169 = property on="Encoder Steps/º" class="DigNum (strict)"("Disabled"=w372) -> ()  [unwired: 2 in, 2 out]
        n170 = property on="Disconnect Motor" class="Bool (strict)"("Disabled"=w372) -> ()  [unwired: 2 in, 2 out]
        n171 = property on="Jog Angle (º)" class="DigNum (strict)"("Disabled"=w372) -> ()  [unwired: 2 in, 2 out]
        n172 = property on="Backward" class="Bool (strict)"("Disabled"=w372) -> ()  [unwired: 2 in, 2 out]
        n173 = property on="Forward" class="Bool (strict)"("Disabled"=w372) -> ()  [unwired: 2 in, 2 out]
        n174 = Enqueue Element(queue=w376, element=rotatory_motor_states."Idle", error in (no error)=w375) -> (error out=w374:errorcluster)  [unwired: 1 in, 2 out]
      }
      frame "Connect Motor" {
        n175 = call "init_Elliptec_VISA_connection.vi"("VISA resource name"=w389) -> ("error out"=w384:errorcluster)  [unwired: 9 in, 1 out]
        n176 = local read "Camera Ready"() -> (w380:bool)
        n177 = Equal?(x=w384, y=errorcluster {"status"=FALSE, "code"=0, "source"=""}) -> (x = y?=w382:T7)
        n178 = Unbundle By Name(w382) -> ("status"=w379:bool)  [unwired: 2 out]
        n179 = And(x=w380, y=w379) -> (x .and. y?=w381:bool)
        n180 = case shown="True" w381 {
          frame False {
          }
          frame True {
            w390 = u8 0 ("Disabled")
            n181 = property on="Calibrate QWP" class="Bool (strict)"("Disabled"=w390) -> ()  [unwired: 2 in, 2 out]
            n182 = property on="Measure Stokes" class="Bool (strict)"("Disabled"=w390) -> ()  [unwired: 2 in, 2 out]
          }
        }
        n183 = local write "Motor Ready"(w379) -> ()
        n184 = case shown="True" w379 {
          frame False {
          }
          frame True {
            w391 = u8 0 ("Disabled")
            n185 = property on="Forward" class="Bool (strict)"("Disabled"=w391) -> ()  [unwired: 2 in, 2 out]
            n186 = property on="Disconnect Motor" class="Bool (strict)"("Disabled"=w391) -> ()  [unwired: 2 in, 2 out]
            n187 = property on="Encoder Steps/º" class="DigNum (strict)"("Disabled"=w391) -> ()  [unwired: 2 in, 2 out]
            n188 = property on="Backward" class="Bool (strict)"("Disabled"=w391) -> ()  [unwired: 2 in, 2 out]
            n189 = property on="Jog Angle (º)" class="DigNum (strict)"("Disabled"=w391) -> ()  [unwired: 2 in, 2 out]
          }
        }
        n190 = Enqueue Element(queue=w388, element=rotatory_motor_states."Set Jog Step", error in (no error)=w387) -> (error out=w385:errorcluster)  [unwired: 1 in, 2 out]
      }
      frame "Stop All" {
        n191 = VISA Close(VISA resource name=w394) -> ()  [unwired: 1 in, 1 out]
        n192 = local write "Motor Ready"(FALSE) -> ()
      }
      frame "Idle", Default {
      }
      frame "Move Forward" {
        n193 = call "move_forward.vi"("Motor \"Name\""=w401, "VISA resource name"=w402) -> ()  [unwired: 8 in, 2 out]
        n194 = Enqueue Element(queue=w399, element=rotatory_motor_states."Idle", error in (no error)=w398) -> (error out=w397:errorcluster)  [unwired: 1 in, 2 out]
      }
      frame "Move Backward" {
        n195 = call "move_backwards.vi"("Motor \"Name\""=w407, "VISA resource name"=w408) -> ()  [unwired: 8 in, 2 out]
        n196 = Enqueue Element(queue=w403, element=rotatory_motor_states."Idle", error in (no error)=w405) -> (error out=w404:errorcluster)  [unwired: 1 in, 2 out]
      }
    }
  }
  n197 = Release Queue(queue=w32, error in (no error)=w31) -> ()  [unwired: 1 in, 3 out]
  n198 = local write "Calibrate QWP"(w18) -> ()
  n199 = local write "Live"(w18) -> ()
  n200 = local write "Measure Stokes"(w18) -> ()
  n201 = property on="Camera Properties" class="Bool (strict)"("Disabled"=w19) -> ()  [unwired: 2 in, 2 out]
  n202 = property on="Calibrate QWP" class="Bool (strict)"("Disabled"=w19) -> ()  [unwired: 2 in, 2 out]
  n203 = property on="Live" class="Bool (strict)"("Disabled"=w19) -> ()  [unwired: 2 in, 2 out]
  n204 = property on="Measure Stokes" class="Bool (strict)"("Disabled"=w19) -> ()  [unwired: 2 in, 2 out]
  n205 = property on="Disconnect Camera" class="Bool (strict)"("Disabled"=w19) -> ()  [unwired: 2 in, 2 out]
  n206 = property on="Grab Image" class="Bool (strict)"("Disabled"=w19) -> ()  [unwired: 2 in, 2 out]
  n207 = Obtain Queue(name (unnamed)="Camera State", element data type=states_camera."Idle", error in (no error)=errorcluster {"status"=FALSE, "code"=0, "source"=""}) -> (queue out=w38:refnum<queue>, error out=w37:errorcluster)  [unwired: 2 in, 1 out]
  "Camera State Queue" <- w38
  n208 = while {
    tunnel: w38 -> [w414]
    tunnel: w37 -> [w413]
    tunnel: [w412] -> w42
    tunnel: [w411] -> w40
    stop <- w410 stop-if-true
    n209 = event shown="[8] \"Calibrate QWP\": Value Change" {
      selector: _ -> [_ _ _ _ _ _ _ _ _]
      dyn-events: _ -> [_ _ _ _ _ _ _ _ _]
      timeout: _ -> [_ _ _ _ _ _ _ _ _]
      tunnel: w414 -> [_ w419 w424 w429 w434 w439 w444 w450 w455]
      tunnel: w413 -> [_ w418 w423 w428 w433 w438 w443 w449 w454]
      tunnel: [_ w417 w422 w427 w432 w436 w441 w447 w452] -> w412
      tunnel: [_ w416 w421 w426 w431 w437 w442 w448 w453] -> w411
      tunnel: [_ _ _ _ _ _ TRUE _ _] -> w410
      event Timeout {
        n210 = event-data() -> ()  [unwired: 1 in, 1 out]
      }
      event "Grab Image": Value Change {
        n211 = event-data() -> ()  [unwired: 1 in, 1 out]
        n212 = Enqueue Element(queue=w419, element=states_camera."Grab Image", error in (no error)=w418) -> (queue out=w417:refnum<queue>, error out=w416:errorcluster)  [unwired: 1 in, 1 out]
      }
      event "Connect Camera": Value Change {
        n213 = event-data() -> ()  [unwired: 1 in, 1 out]
        n214 = Enqueue Element(queue=w424, element=states_camera."Init Camera", error in (no error)=w423) -> (queue out=w422:refnum<queue>, error out=w421:errorcluster)  [unwired: 1 in, 1 out]
      }
      event "Live": Value Change {
        n215 = event-data() -> ()  [unwired: 1 in, 1 out]
        n216 = Enqueue Element(queue=w429, element=states_camera."Set Live", error in (no error)=w428) -> (queue out=w427:refnum<queue>, error out=w426:errorcluster)  [unwired: 1 in, 1 out]
      }
      event "Camera Properties": Value Change {
        n217 = event-data() -> ()  [unwired: 1 in, 1 out]
        n218 = Enqueue Element(queue=w434, element=states_camera."Open Properties", error in (no error)=w433) -> (queue out=w432:refnum<queue>, error out=w431:errorcluster)  [unwired: 1 in, 1 out]
      }
      event "Disconnect Camera": Value Change {
        n219 = event-data() -> ()  [unwired: 1 in, 1 out]
        n220 = Enqueue Element(queue=w439, element=states_camera."Disconnect Camera", error in (no error)=w438) -> (queue out=w436:refnum<queue>, error out=w437:errorcluster)  [unwired: 1 in, 1 out]
      }
      event "Stop All": Value Change {
        n221 = event-data() -> ()  [unwired: 1 in, 1 out]
        n222 = Enqueue Element(queue=w444, element=states_camera."Stop Program", error in (no error)=w443) -> (queue out=w441:refnum<queue>, error out=w442:errorcluster)  [unwired: 1 in, 1 out]
      }
      event "Measure Stokes": Value Change {
        n223 = event-data() -> ()  [unwired: 1 in, 6 out]
        n224 = Enqueue Element(queue=w450, element=states_camera."Measure Stokes", error in (no error)=w449) -> (queue out=w447:refnum<queue>, error out=w448:errorcluster)  [unwired: 1 in, 1 out]
      }
      event "Calibrate QWP": Value Change {
        n225 = event-data() -> ()  [unwired: 1 in, 6 out]
        n226 = Enqueue Element(queue=w455, element=states_camera."Calibrate QWP Position", error in (no error)=w454) -> (queue out=w452:refnum<queue>, error out=w453:errorcluster)  [unwired: 1 in, 1 out]
      }
    }
    n227 = Wait (ms)(milliseconds to wait=u32 50) -> ()  [unwired: 1 out]
  }
  n228 = String To Path(string="C:\\Users\\laboratori\\Desktop\\PySLM_VeReady\\pyVeReady\\polarization_analysis\\experimental_characterization\\gui_obtained_measures") -> (path=w1:path)
  n229 = String To Path(string="C:\\Users\\laboratori\\Desktop\\PySLM_VeReady\\pyVeReady\\utils\\image_utils.py") -> (path=w3:path)
  n230 = while {
    tunnel: w38 -> [w466]
    tunnel: w37 -> [w465]
    tunnel: "ICImagingControl" -> [w463]
    tunnel: [w462] -> w41
    tunnel: w1 -> [w458]
    tunnel: w9 -> [w457]
    tunnel: w3 -> [w456]
    stop <- w459 stop-if-true
    n231 = Dequeue Element(queue=w466, error in (no error)=w465) -> (queue out=w460:refnum<queue>, element=w464:T4, error out=w461:errorcluster)  [unwired: 1 in, 1 out]
    n232 = case shown="\"Measure Stokes\"" w464 {
      tunnel: w463 -> [w469 _ w488 w495 w506 w515 w521 w534 w575 _]
      tunnel: [w471 w482 w485 w492 w499 w511 w519 w545 w571 w637] -> w462
      tunnel: w461 -> [w472 w482 w486 w493 w500 w512 w519 w546 w571 w637]
      tunnel: w460 -> [w470 _ w487 w491 w498 w513 _ w544 _ _]
      tunnel: [_ _ _ _ _ _ TRUE _ _ _] -> w459
      tunnel: w458 -> [_ _ _ _ _ _ _ w532 _ _]
      tunnel: w457 -> [_ _ _ _ _ _ _ w530 _ _]
      tunnel: w456 -> [_ _ _ _ _ _ _ w529 _ _]
      frame "Init Camera", Default {
        n233 = flat-sequence {
          tunnel: w469 -> [w473]
          tunnel: [w476] -> w467
          tunnel: w467 -> [w479]
          frame #0 {
            n234 = call <userlib>:"IC_RestoreState.vi"("Color"=FALSE, "ICImagingControl"=w473) -> ()  [unwired: 2 in, 2 out]
          }
          frame #1 {
            w475 = u8 0 ("Disabled")
            n235 = property on="Camera Properties" class="Bool (strict)"("Disabled"=w475) -> ()  [unwired: 2 in, 2 out]
            n236 = property on="Live" class="Bool (strict)"("Disabled"=w475) -> ()  [unwired: 2 in, 2 out]
            n237 = property on="Disconnect Camera" class="Bool (strict)"("Disabled"=w475) -> ()  [unwired: 2 in, 2 out]
            n238 = property on="Grab Image" class="Bool (strict)"("Disabled"=w475) -> ()  [unwired: 2 in, 2 out]
          }
          frame #2 {
            w476 = TRUE
            n239 = local write "Connect Camera"(FALSE) -> ()
            n240 = local write "Camera Ready"(w476) -> ()
          }
          frame #3 {
            n241 = local read "Motor Ready"() -> (w480:bool)
            n242 = And(x=w480, y=w479) -> (x .and. y?=w478:bool)
            n243 = case shown="True" w478 {
              frame False {
              }
              frame True {
                w481 = u8 0 ("Disabled")
                n244 = property on="Measure Stokes" class="Bool (strict)"("Disabled"=w481) -> ()  [unwired: 2 in, 2 out]
                n245 = property on="Calibrate QWP" class="Bool (strict)"("Disabled"=w481) -> ()  [unwired: 2 in, 2 out]
              }
            }
          }
        }
        n246 = Enqueue Element(queue=w470, element=states_camera."Idle", error in (no error)=w472) -> (error out=w471:errorcluster)  [unwired: 1 in, 2 out]
      }
      frame "Idle" {
      }
      frame "Open Properties" {
        n247 = invoke class="IICImagingControl" method="ShowPropertyDialog"(reference=w488) -> ()  [unwired: 2 in, 3 out]
        n248 = Enqueue Element(queue=w487, element=states_camera."Idle", error in (no error)=w486) -> (error out=w485:errorcluster)  [unwired: 1 in, 2 out]
        n249 = local write "Camera Properties"(FALSE) -> ()
      }
      frame "Grab Image" {
        w490 = FALSE
        n250 = call <userlib>:"IC_Grab_IMAQ.vi"("ICImagingControl In"=w495) -> ("Image Out"=→"Snapped Image":T2)  [unwired: 2 in, 3 out]
        n251 = Enqueue Element(queue=w491, element=states_camera."Idle", error in (no error)=w493) -> (error out=w492:errorcluster)  [unwired: 1 in, 2 out]
        n252 = local write "Grab Image"(w490) -> ()
        n253 = local write "Live"(w490) -> ()
      }
      frame "Disconnect Camera" {
        w496 = u8 2 ("Disabled")
        w503 = FALSE
        n254 = property class="IICImagingControl"(reference=w506) -> (reference out=w504:refnum<k7>, "LiveVideoRunning"=w505:bool)  [unwired: 1 in, 1 out]
        n255 = local write "Disconnect Camera"(w503) -> ()
        n256 = local write "Camera Ready"(w503) -> ()
        n257 = case shown="True" w505 {
          tunnel: w504 -> [w507 w509]
          tunnel: [w507 w508] -> w501
          frame False {
          }
          frame True {
            n258 = invoke class="IICImagingControl" method="LiveStop"(reference=w509) -> (reference out=w508:refnum<k7>)  [unwired: 2 in, 2 out]
          }
        }
        n259 = Enqueue Element(queue=w498, element=states_camera."Idle", error in (no error)=w500) -> (error out=w499:errorcluster)  [unwired: 1 in, 2 out]
        n260 = property class="IICImagingControl"(reference=w501, "Device"="") -> ()  [unwired: 1 in, 2 out]
        n261 = property on="Camera Properties" class="Bool (strict)"("Disabled"=w496) -> ()  [unwired: 2 in, 2 out]
        n262 = property on="Live" class="Bool (strict)"("Disabled"=w496) -> ()  [unwired: 2 in, 2 out]
        n263 = property on="Disconnect Camera" class="Bool (strict)"("Disabled"=w496) -> ()  [unwired: 2 in, 2 out]
        n264 = property on="Grab Image" class="Bool (strict)"("Disabled"=w496) -> ()  [unwired: 2 in, 2 out]
        n265 = property on="Measure Stokes" class="Bool (strict)"("Disabled"=w496) -> ()  [unwired: 2 in, 2 out]
      }
      frame "Set Live" {
        n266 = local read "Live"() -> (w514:bool)
        n267 = case shown="True" w514 {
          tunnel: w515 -> [w516 w517]
          frame False {
            n268 = invoke class="IICImagingControl" method="LiveStop"(reference=w516) -> ()  [unwired: 2 in, 3 out]
          }
          frame True {
            n269 = invoke class="IICImagingControl" method="LiveStart"(reference=w517) -> ()  [unwired: 2 in, 3 out]
          }
        }
        n270 = Enqueue Element(queue=w513, element=states_camera."Idle", error in (no error)=w512) -> (error out=w511:errorcluster)  [unwired: 1 in, 2 out]
      }
      frame "Stop Program" {
        w518 = FALSE
        n271 = property class="IICImagingControl"(reference=w521) -> (reference out=w524:refnum<k7>, "LiveVideoRunning"=w523:bool)  [unwired: 1 in, 1 out]
        n272 = case shown="False" w523 {
          tunnel: w524 -> [w526 w528]
          tunnel: [w526 w527] -> w525
          frame False {
          }
          frame True {
            n273 = invoke class="IICImagingControl" method="LiveStop"(reference=w528) -> (reference out=w527:refnum<k7>)  [unwired: 2 in, 2 out]
          }
        }
        n274 = property class="IICImagingControl"(reference=w525, "Device"="") -> ()  [unwired: 1 in, 2 out]
        n275 = local write "Camera Ready"(w518) -> ()
        n276 = local write "Live"(w518) -> ()
      }
      frame "Measure Stokes" {
        w541 = TRUE
        n277 = local read "Motor Ready"() -> (w543:bool)
        n278 = local read "Camera Ready"() -> (w542:bool)
        n279 = local read "Encoder Steps/º"() -> (w536:i32)
        n280 = local read "VISA Rotatory Motor"() -> (w537:refnum<visa-resource-name>)
        n281 = local read "Motor Name"() -> (w535:string)
        n282 = local read "N Angles"() -> (w531:i16)
        n283 = Equal?(x=w543, y=w541) -> (x = y?=w540:bool)
        n284 = Equal?(x=w542, y=w541) -> (x = y?=w539:bool)
        n285 = And(x=w540, y=w539) -> (x .and. y?=w538:bool)
        n286 = case shown="True" w538 {
          tunnel: w537 -> [_ w564]
          tunnel: w536 -> [_ w558]
          tunnel: w535 -> [_ w550]
          tunnel: w534 -> [_ w555]
          tunnel: [_ FALSE] -> w533
          tunnel: w532 -> [_ w554]
          tunnel: w531 -> [_ w557]
          tunnel: w530 -> [_ w552]
          tunnel: w529 -> [_ w551]
          frame False {
          }
          frame True {
            n287 = Divide(x=180.0, y=w557) -> (x/y=w559:dbl)
            n288 = local write "Jog Angle (º)"(w559) -> ()
            n289 = local read "Modulation Mode Double Pass"() -> (w553:string)
            n290 = call "set_jog_step.vi"("Motor \"Name\""=w550, "Encoder Pulses per Degree"=w558, "Degrees"=w559, "VISA resource name"=w564) -> ("error out"=w562:errorcluster, "VISA resource name out"=w563:refnum<visa-resource-name>)  [unwired: 5 in]
            n291 = call "go_home.vi"("error in (no error)"=w562, "Motor \"Name\""=w550, "VISA resource name"=w563) -> ("VISA resource name out"=w549:refnum<visa-resource-name>)  [unwired: 7 in, 1 out]
            n292 = flat-sequence {
              tunnel: [w566] -> w548
              tunnel: w549 -> [w566]
              frame #0 {
                n293 = Wait (ms)(milliseconds to wait=u32 500) -> ()  [unwired: 1 out]
              }
            }
            n294 = call "averaged_stokes_acquisition_single_tiff.vi"("Motor \"Name\""=w550, "Beam Type"=w553, "VISA resource name"=w548, "Encoder Pulses per Degree"=w558, "Number of Angles"=w557, "Number of Measures"=10, "ICImagingControl In"=w555, "session in"=w552, "Saving Path"=w554, "module path"=w551) -> ()  [unwired: 6 in]
          }
        }
        n295 = Enqueue Element(queue=w544, element=states_camera."Idle", error in (no error)=w546) -> (error out=w545:errorcluster)  [unwired: 1 in, 2 out]
        n296 = local write "Measure Stokes"(w533) -> ()
      }
      frame "Calibrate QWP Position" {
        n297 = local read "Degree Sampling"() -> (w567:dbl)
        n298 = local read "VISA Rotatory Motor"() -> (w574:refnum<visa-resource-name>)
        n299 = local read "Camera Ready"() -> (w579:bool)
        n300 = local read "Motor Ready"() -> (w580:bool)
        n301 = local read "Encoder Steps/º"() -> (w572:i32)
        n302 = local read "Motor Name"() -> (w573:string)
        n303 = And(x=w580, y=w579) -> (x .and. y?=w578:bool)
        n304 = Quotient & Remainder(x=135.0, y=w567) -> (floor(x/y)=w576:dbl)  [unwired: 1 out]
        n305 = Initialize Array(0.0, 0 ("dimension size")) -> (w568:dbl[])
        n306 = case shown="True" w578 {
          selector: w578 -> [_ w587]
          tunnel: w576 -> [_ w608]
          tunnel: w575 -> [_ w607]
          tunnel: w574 -> [_ w600]
          tunnel: w573 -> [_ w601]
          tunnel: w567 -> [_ w602]
          tunnel: w572 -> [_ w589]
          tunnel: w568 -> [_ w596]
          tunnel: w567 -> [_ w595]
          frame False {
          }
          frame True {
            # "Max"
            n307 = for {
              N: w608 -> [_]
              tunnel: w607 -> [w626]
              shift-right: [w622] -> w593
              shift-left: w596 -> [w624]
              tunnel: w582 -> [w621]
              tunnel: w588 -> [w620]
              tunnel: w590 -> [w619]
              shift-right: [w615] -> w594
              shift-left: w596 -> [w618]
              tunnel: w595 -> [w617]
              tunnel: [w613] -> w586
              tunnel: w587 -> [w613]
              i -> [w614]
              n308 = flat-sequence {
                tunnel: w626 -> [w628]
                tunnel: [w627] -> w625
                tunnel: w625 -> [w632]
                tunnel: [w631] -> w623
                tunnel: w621 -> [w635]
                tunnel: w620 -> [w634]
                tunnel: w619 -> [w633]
                frame #0 {
                  n309 = call <userlib>:"IC_Grab_IMAQ.vi"("ICImagingControl In"=w628) -> ("Image Out"=w627:T2)  [unwired: 2 in, 3 out]
                }
                frame #1 {
                  n310 = call "IMAQ ImageToArray"("Image"=w632) -> ("Image Pixels (U8)"=w630:u8[][])  [unwired: 3 in, 4 out]
                  n311 = To Double Precision Float(number=w630) -> (double precision float=w629:dbl[][])
                  n312 = Add Array Elements(numeric array=w629) -> (sum=w631:dbl)
                }
                frame #2 {
                  n313 = call "move_forward.vi"("error in (no error)"=w633, "Motor \"Name\""=w635, "VISA resource name"=w634) -> ()  [unwired: 7 in, 2 out]
                }
                frame #3 {
                  n314 = Wait (ms)(milliseconds to wait=u32 100) -> ()  [unwired: 1 out]
                }
              }
              n315 = Multiply(x=w614, y=w617) -> (x*y=w616:dbl)
              n316 = Build Array (concatenate)(w618, w616) -> (w615:dbl[])
              n317 = Build Array (concatenate)(w624, w623) -> (w622:dbl[])
            }
            n318 = call "set_home_offset.vi"("Motor \"Name\""=w601, "Encoder Pulses per Degree"=w589, "Degrees"=0.0, "VISA resource name"=w600) -> ("error out"=w599:errorcluster, "VISA resource name out"=w598:refnum<visa-resource-name>)  [unwired: 6 in]
            n319 = call "set_jog_step.vi"("Motor \"Name\""=w601, "error in (no error)"=w599, "Encoder Pulses per Degree"=w589, "Degrees"=w602, "VISA resource name"=w598) -> ("error out"=w605:errorcluster, "VISA resource name out"=w606:refnum<visa-resource-name>)  [unwired: 4 in]
            n320 = local write "Jog Angle (º)"(w602) -> ()
            n321 = call "go_home.vi"("error in (no error)"=w605, "Motor \"Name\""=w601, "VISA resource name"=w606) -> ("error out"=w603:errorcluster, "VISA resource name out"=w604:refnum<visa-resource-name>)  [unwired: 7 in]
            n322 = flat-sequence {
              tunnel: [w611] -> w582
              tunnel: w601 -> [w611]
              tunnel: [w610] -> w588
              tunnel: w604 -> [w610]
              tunnel: [w609] -> w590
              tunnel: w603 -> [w609]
              frame #0 {
                n323 = Wait (ms)(milliseconds to wait=u32 1000) -> ()  [unwired: 1 out]
              }
            }
            n324 = Not(x=w586) -> (.not. x?=w585:bool)
            n325 = Array Max & Min(array=w593) -> (max index (indices)=w581:i32)  [unwired: 3 out]
            n326 = Bundle(w594, w593) -> (→"?":cluster{dbl[], dbl[]})  [unwired: 1 in]
            n327 = local write "Calibrate QWP"(w585) -> ()
            n328 = Multiply(x=w581, y=w602) -> (x*y=w591:dbl)
            n329 = call "set_home_offset.vi"("Motor \"Name\""=w582, "error in (no error)"=w590, "Encoder Pulses per Degree"=w589, "Degrees"=w591, "VISA resource name"=w588) -> ("error out"=w583:errorcluster, "VISA resource name out"=w584:refnum<visa-resource-name>)  [unwired: 5 in]
            n330 = call "go_home.vi"("error in (no error)"=w583, "Motor \"Name\""=w582, "VISA resource name"=w584) -> ()  [unwired: 7 in, 2 out]
          }
        }
      }
      frame "Calibrate SLM Phase Modulation" {
        n331 = flat-sequence {
          frame #0 {
            n332 = local write "Modulation Type Single Pass"("Calibration") -> ()
          }
          frame #1 {
            n333 = for {
              N: 256 -> [_]
              i -> [w640]
              n334 = flat-sequence {
                tunnel: w640 -> [w642]
                frame #0 {
                  n335 = local write "Multipurpose\nCoefficient"(w642) -> ()
                  n336 = Wait (ms)(milliseconds to wait=u32 200) -> ()  [unwired: 1 out]
                }
                frame #1 {
                  n337 = while {
                    tunnel: [200] -> w643
                    stop <- w645 stop-if-true
                    n338 = local read "Signal Ready"() -> (w645:bool)
                  }
                  n339 = Wait (ms)(milliseconds to wait=w643) -> ()  [unwired: 1 out]
                }
                frame #2 {
                }
              }
            }
          }
        }
      }
    }
  }
  n340 = Merge Errors(w40, w41) -> (w39:errorcluster)
  n341 = Release Queue(queue=w42, error in (no error)=w39) -> ()  [unwired: 1 in, 3 out]
  "SLM Ready" <- FALSE
  "Motor Ready" <- FALSE
  "Camera Ready" <- FALSE
  "Signal Ready" <- FALSE
